vi "Read Data.vi"(8 "error in (no error)":errorcluster, 11 "File Data Message in":refnum<class "File Data Message.lvclass">) -> (0 "error out":errorcluster, 2 "Base Data Lib:Data":refnum<class "Data.lvclass">, 3 "File Data Message out":refnum<class "File Data Message.lvclass">)   [LabVIEW 2016, in "File Library.lvlib" / "File Data Message.lvclass"]
uses:
  File Data Message.lvclass
  <vilib>/MSR Consulting, LLC/General Reuse/Data/Data.lvclass
  File Data Message.lvclass/File Data Message.ctl
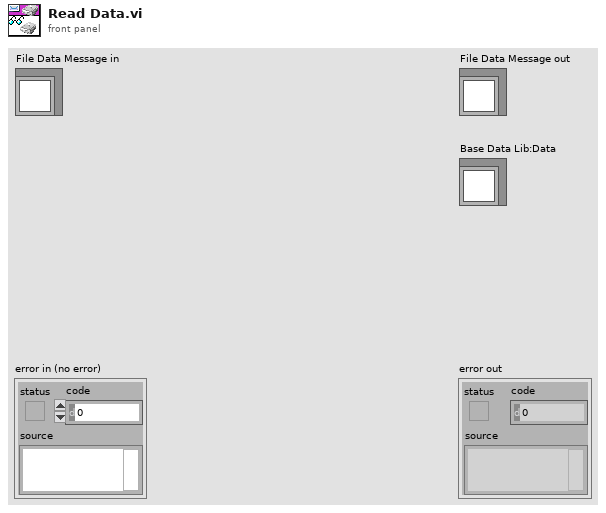
[diagram p1: front panel]
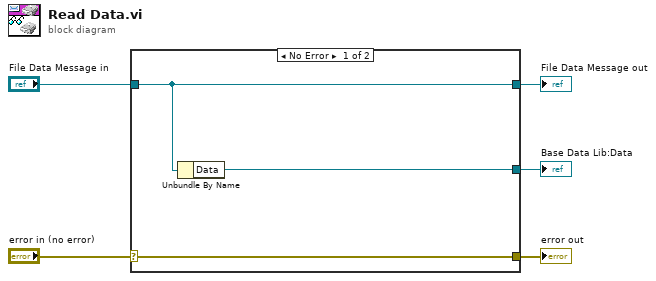
[diagram p0: block diagram]
diagram:
  n1 = case shown="No Error" "error in (no error)" {
    selector: "error in (no error)" -> [w8 w9]
    tunnel: [w8 w9] -> w4
    tunnel: [w7 w10] -> w2
    tunnel: "File Data Message in" -> [w7 w10]
    tunnel: [w6 _] -> w1
    frame No Error {
      n2 = Unbundle By Name(w7) -> ("Data"=w6:refnum<class "Data.lvclass">)
    }
    frame Error {
    }
  }
  "error out" <- w4
  "File Data Message out" <- w2
  "Base Data Lib:Data" <- w1
